vi "Move 2D and Wait.vi"(4 "error IO":errorcluster, 6 "Position table":dbl[](array[numeric])) -> (0 "error out":errorcluster)   [LabVIEW 2010, in "PI E710 Stage.lvlib"]
uses:
  PI E710 Stage.lvlib
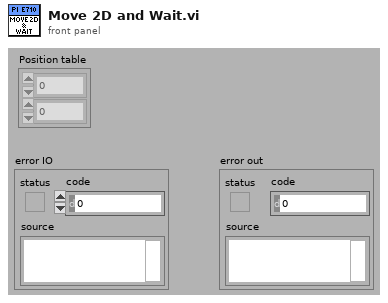
[diagram p1: front panel]
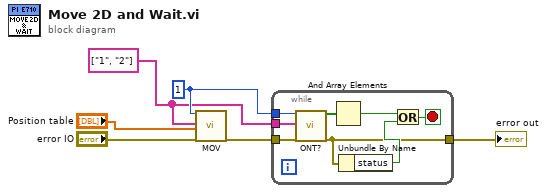
[diagram p0: block diagram]
diagram:
  w2 = string[] ["1", "2"] ("Axes to move")
  w4 = 1 ("System no.")
  n1 = call "MOV.vi"("System no."=w4, "Axes to move"=w2, "Position values"="Position table", "error in"="error IO") -> ("error out"=w5:errorcluster)  [unwired: 15 in]
  n2 = while {
    tunnel: w5 -> [w14]
    tunnel: w4 -> [w13]
    tunnel: w2 -> [w12]
    tunnel: [w7] -> w3
    stop <- w10 stop-if-true
    n3 = call "ONT?.vi"("System no."=w13, "Axes to query"=w12, "error in"=w14) -> ("Axis on target?"=w11:bool[], "error out"=w7:errorcluster)  [unwired: 15 in]
    n4 = And Array Elements(Boolean array=w11) -> (logical AND=w9:bool)
    n5 = Unbundle By Name(w7) -> ("status"=w8:bool)
    n6 = Or(x=w9, y=w8) -> (x .or. y?=w10:bool)
  }
  "error out" <- w3
